vi "Read Packets.vi"(11 "PacketCollection in":refnum<class "PacketCollection.lvclass">) -> (2 "Packets":refnum<class "ControlPacket.lvclass">[](array[class]), 3 "PacketCollection out":refnum<class "PacketCollection.lvclass">)   [LabVIEW 2013, in "MQTT Server.lvlib" / "PacketCollection.lvclass"]
uses:
  PacketCollection.lvclass
  <vilib>/LabVIEW Open Source Project/MQTT Control Packets/Control Packets/ControlPacket/ControlPacket.lvclass
  PacketCollection.lvclass/PacketCollection.ctl
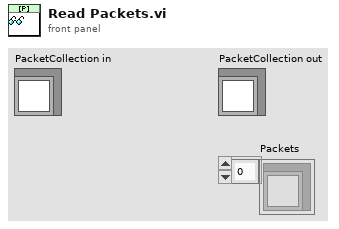
[diagram p1: front panel]
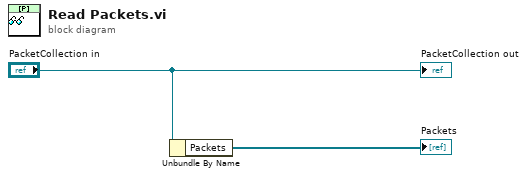
[diagram p0: block diagram]
diagram:
  n1 = Unbundle By Name("PacketCollection in") -> ("Packets"=→"Packets":refnum<class "ControlPacket.lvclass">[])
  "PacketCollection out" <- "PacketCollection in"
